vi "Operations queue.vi"(8 "error in":errorcluster, 11 "queue in":refnum<queue>) -> (0 "error out":errorcluster, 1 "Operations Queued This Loop":cluster{"Source":T1, "Command":string}[](array[cluster]), 2 "Set Times of Operations Queued This Loop":timestamp[](array[timestamp]), 3 "queue out":refnum<queue>)   [LabVIEW 2018]
uses:
  Event Sources.ctl
  CAEN globals.vi
  <userlib>/_OpenG.lib/array/array.llb/Search 1D Array (Boolean)__ogtk.vi
  <userlib>/_OpenG.lib/array/array.llb/Sort 1D Array (I32)__ogtk.vi
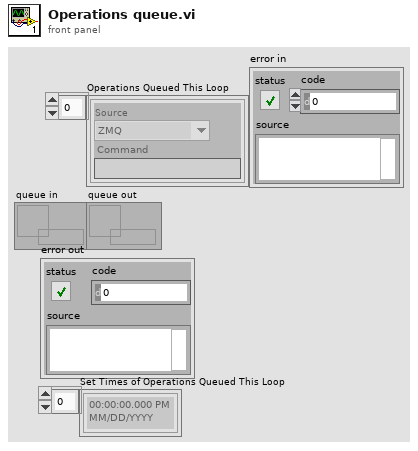
[diagram p1: front panel]
types:
  T1 = typedef "Event Sources.ctl" = enum16{"ZMQ", "INTERNAL", "Check_Errors", "Send_ZMQ_Reply", "Save_PMT_Voltages", "Set_Ramp_Voltage", "Restore PMT Voltages"}
  T2 = cluster{"seconds since 1Jan1904":timestamp, "element":cluster{"Source":T1, "Command":string}}[]
  T3 = cluster{"seconds since 1Jan1904":timestamp, "element":cluster{"Source":T1, "Command":string}}
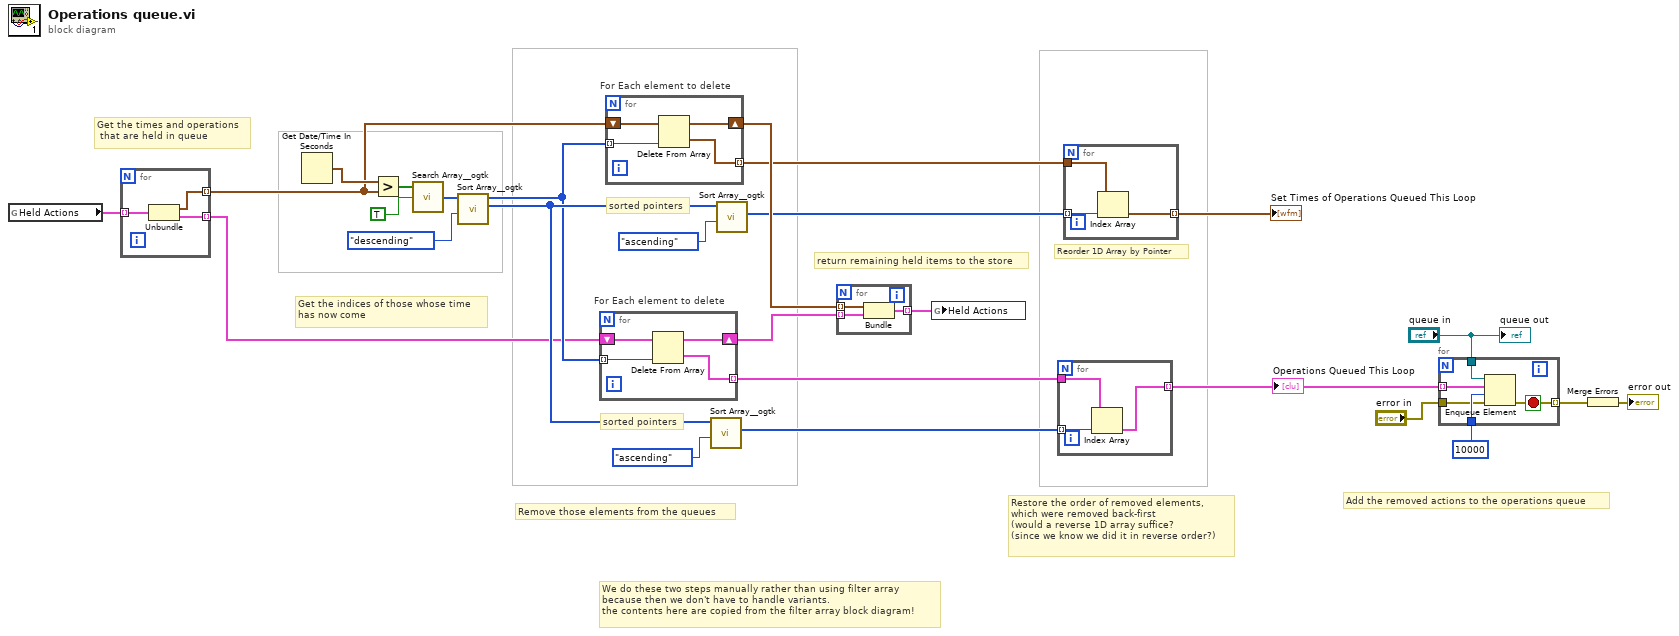
[diagram p0: block diagram]
diagram:
  # "return remaining held items to the store"
  # "Restore the order of removed elements,\nwhich were removed back-first\n(would a reverse 1D array suffice?\n(since we know we did it in reverse order?)"
  # "We do these two steps manually rather than using filter array\nbecause then we don't have to handle variants.\nthe contents here are copied from the filter array block diagram!"
  # "Remove those elements from the queues"
  # "Get the indices of those whose time\nhas now come"
  # "Get the times and operations\n that are held in queue"
  # "sorted pointers"
  # "Reorder 1D Array by Pointer"
  # "sorted pointers"
  # "Add the removed actions to the operations queue"
  n1 = global read "CAEN globals.vi" "Held Actions"() -> (w3:T2)
  n2 = for {
    tunnel: w3 -> [w29] mode=indexing
    tunnel: [w28] -> w2 mode=indexing
    tunnel: [w27] -> w1 mode=indexing
    n3 = Unbundle(w29) -> ("seconds since 1Jan1904"=w28:timestamp, "element"=w27:cluster{"Source":T1, "Command":string})
  }
  n4 = Get Date/Time In Seconds() -> (seconds since 1Jan1904=w16:timestamp)
  n5 = Greater?(x=w16, y=w2) -> (0:w15:bool[])
  n6 = call-poly <userlib>:"Search Array__ogtk.vi"("Array"=w15, "Element Data"=TRUE) -> ("Indices of Elements"=w12:i32[])  [unwired: 7 in]
  n7 = call-poly <userlib>:"Sort Array__ogtk.vi"("Order"=enum16{"ascending", "descending"}."descending", "Array in"=w12) -> ("Sorted Pointers"=w5:i32[], "Sorted Array out"=w4:i32[])  [unwired: 8 in]
  n8 = for "For Each element to delete" {
    tunnel: w4 -> [w33] mode=indexing
    shift-right: [w32] -> w18
    shift-left: w1 -> [w31]
    tunnel: [w30] -> w7 mode=indexing
    n9 = Delete From Array(array=w31, index=w33) -> (deleted portion=w30:cluster{"Source":T1, "Command":string}, array with subset deleted=w32:cluster{"Source":T1, "Command":string}[])  [unwired: 1 in]
  }
  n10 = for "For Each element to delete" {
    tunnel: w4 -> [w37] mode=indexing
    shift-right: [w36] -> w19
    shift-left: w2 -> [w35]
    tunnel: [w34] -> w11 mode=indexing
    n11 = Delete From Array(array=w35, index=w37) -> (deleted portion=w34:timestamp, array with subset deleted=w36:timestamp[])  [unwired: 1 in]
  }
  n12 = call-poly <userlib>:"Sort Array__ogtk.vi"("Order"=enum16{"ascending", "descending"}."ascending", "Array in"=w5) -> ("Sorted Pointers"=w8:i32[])  [unwired: 8 in, 1 out]
  n13 = call-poly <userlib>:"Sort Array__ogtk.vi"("Order"=enum16{"ascending", "descending"}."ascending", "Array in"=w5) -> ("Sorted Pointers"=w10:i32[])  [unwired: 8 in, 1 out]
  n14 = for {
    tunnel: w19 -> [w40] mode=indexing
    tunnel: w18 -> [w39] mode=indexing
    tunnel: [w38] -> w17 mode=indexing
    n15 = Bundle("seconds since 1Jan1904"=w40, "element"=w39) -> (w38:T3)  [unwired: 1 in]
  }
  n16 = global write "CAEN globals.vi" "Held Actions"(w17) -> ()
  n17 = for {
    tunnel: w7 -> [w43]
    tunnel: [w42] -> w26 mode=indexing
    tunnel: w8 -> [w41] mode=indexing
    n18 = Index Array(array=w43, index=w41) -> (element=w42:cluster{"Source":T1, "Command":string})
  }
  "Operations Queued This Loop" <- w26
  n19 = for {
    tunnel: w11 -> [w46]
    tunnel: [w45] -> w21 mode=indexing
    tunnel: w10 -> [w44] mode=indexing
    n20 = Index Array(array=w46, index=w44) -> (element=w45:timestamp)
  }
  "Set Times of Operations Queued This Loop" <- w21
  n21 = for {
    tunnel: w26 -> [w51] mode=indexing
    tunnel: "queue in" -> [w50]
    tunnel: [w49] -> w24 mode=indexing
    tunnel: 10000 ("timeout in ms (-1)") -> [w48]
    tunnel: "error in" -> [w47]
    stop <- w49 stop-if-true
    n22 = Enqueue Element(queue=w50, element=w51, timeout in ms (-1)=w48, error in (no error)=w47) -> (error out=w49:errorcluster)  [unwired: 2 out]
  }
  n23 = Merge Errors(w24) -> (→"error out":errorcluster)
  "queue out" <- "queue in"
